vi "FTW-XML-Element-Append.vi"(0 "Parent Element":refnum<k20>, 5 "XML Element to Append":string, 11 "error in":errorcluster) -> (4 "Parent Element out":refnum<k20>, 6 "New Element":refnum<k20>, 15 "error out":errorcluster)   [LabVIEW 2015]
uses:
  <resource>/objmgr/DOMUserDefRef.rc
panel:
  # "Inputs"
  # "Outputs"
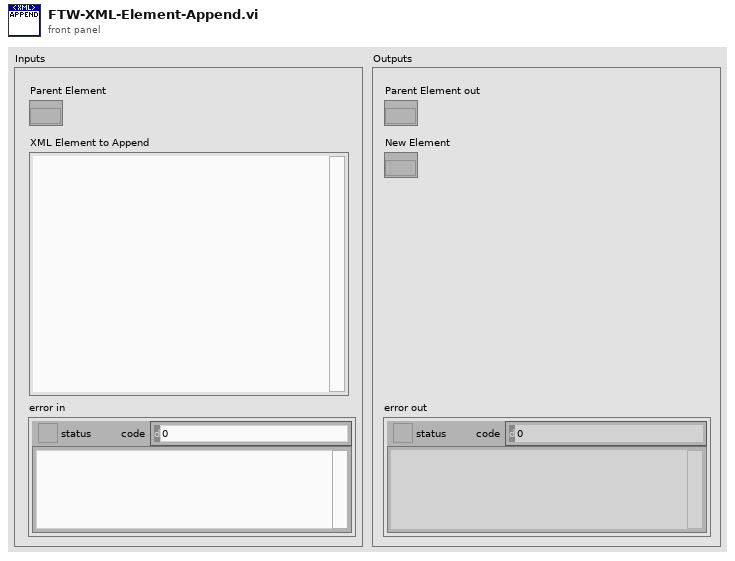
[diagram p1: front panel]
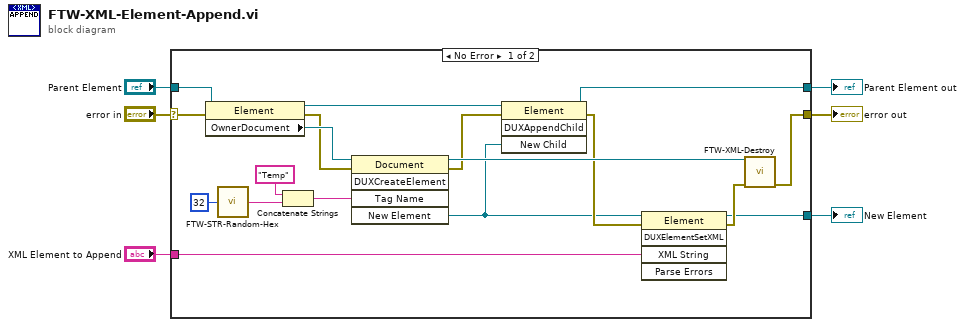
[diagram p0: block diagram]
diagram:
  n1 = case shown="No Error" "error in" {
    selector: "error in" -> [w23 w26]
    tunnel: [w20 w26] -> w6
    tunnel: "Parent Element" -> [w24 w25]
    tunnel: [w21 w25] -> w3
    tunnel: "XML Element to Append" -> [w17 _]
    tunnel: [w7 _] -> w1
    frame No Error {
      n2 = property class="Element"(reference=w24, error in=w23) -> (reference out=w22:refnum<k20>, error out=w18:errorcluster, "OwnerDocument"=w19:refnum<k20>)
      n3 = call "FTW-STR-Random-Hex.vi"("String Length"=32) -> ("Random Hex String"=w13:string)  [unwired: 3 in]
      n4 = Concatenate Strings("Temp" ("string"), w13) -> (w12:string)
      n5 = invoke class="Document" method="DUXCreateElement"(reference=w19, error in=w18, "Tag Name"=w12) -> (reference out=w16:refnum<k20>, error out=w10:errorcluster, "New Element"=w8:refnum<k20>)  [unwired: 2 in, 2 out]
      n6 = invoke class="Element" method="DUXAppendChild"(reference=w22, error in=w10, "New Child"=w8) -> (reference out=w21:refnum<k20>, error out=w9:errorcluster)  [unwired: 1 in, 2 out]
      n7 = invoke class="Element" method="DUXElementSetXML"(reference=w8, error in=w9, "XML String"=w17) -> (reference out=w7:refnum<k20>, error out=w15:errorcluster)  [unwired: 2 in, 3 out]
      n8 = call "FTW-XML-Destroy.vi"("XML Node"=w16, "error in"=w15) -> ("error out"=w20:errorcluster)  [unwired: 13 in]
    }
    frame Error {
    }
  }
  "error out" <- w6
  "Parent Element out" <- w3
  "New Element" <- w1
